vi "Tinius Olsen Output Converter.vi"(8 "error in (no error)":errorcluster, 10 "Data Type (FLOAT)":enum16{"FLOAT", "INT", "BYTE", "SHORT"}(ring), 11 "Data String":string="89C1FC42") -> (0 "error out":errorcluster, 2 "Byte Count":i32=8, 3 "Numeric Conversion - SGL":sgl=126.378)   [LabVIEW 2013]
doc: "This subVI converts ASCII Hex data returned from the Tinius Olsen Model 398 Display device to standard numeric values. Byte reversal is performed within the subVI as appropriate. Only the following data encodings are supported for the 398 Display (Packed Binary Format is not included):\n\nFLOAT = 32-bit (single-precision) floating point number (8 characters),\nINT = 16-bit integer (4 characters),\nBYTE = 8-bit integer (2 characters),\nSHORT = 4-bit integer (1 character).\n\nFor simplicity, all converted values are returned as single precision data type (SGL), even in the case of expected integers. Integer data types are assumed to be unsigned. For more details, please see: people.rit.edu/jdweme/labview/Tinius Olsen Data Conversion.pdf\n\nJohn D. Wellin\nDept. of Mechanical Engineering\nRochester Institute of Technology\nJames E. Gleason Bldg. 09-2014\n76 Lomb Memorial Drive\nRochester, NY 14623-5604\nOffice: 585-475-5223\nFax: 585-475-7710\nEmail: jdweme@rit.edu\nWeb: people.rit.edu/jdweme"
uses:
  <vilib>/regexp/Match Regular Expression.xnode
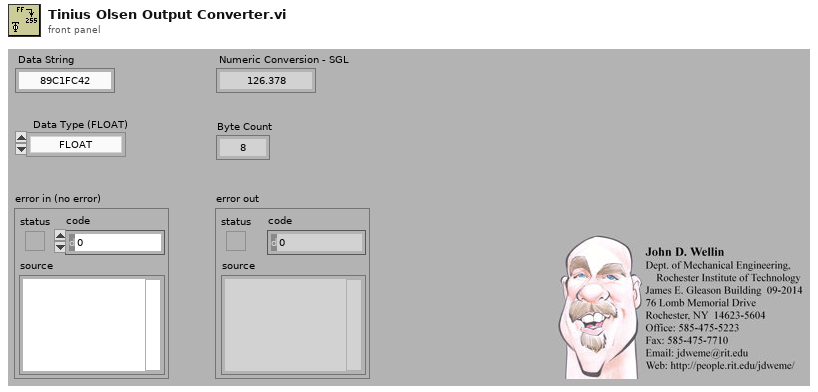
[diagram p1: front panel]
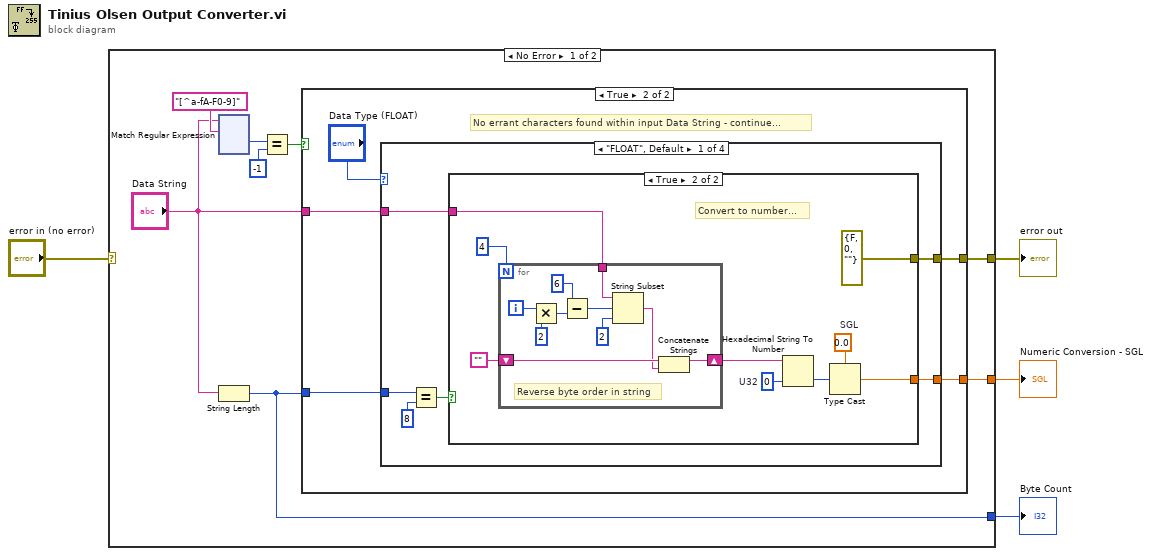
[diagram p0: block diagram]
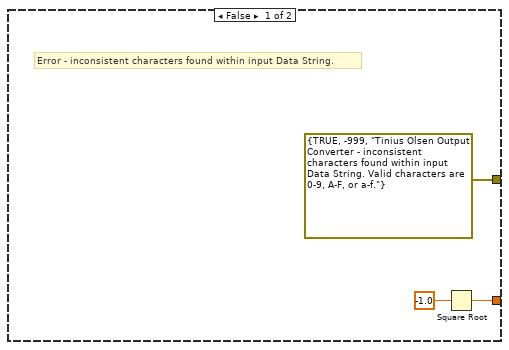
[diagram p2: hidden frame]
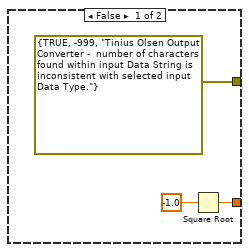
[diagram p3: hidden frame]
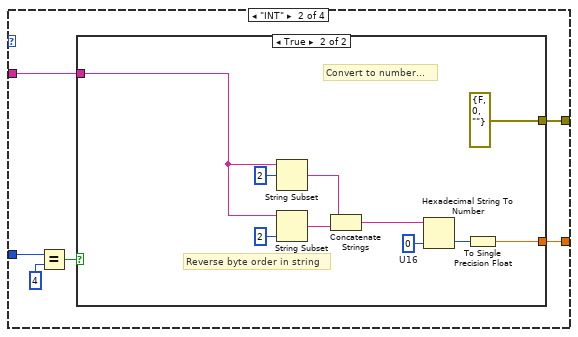
[diagram p4: hidden frame]
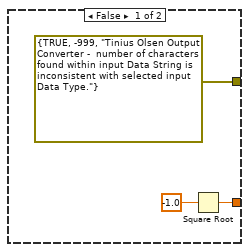
[diagram p5: hidden frame]
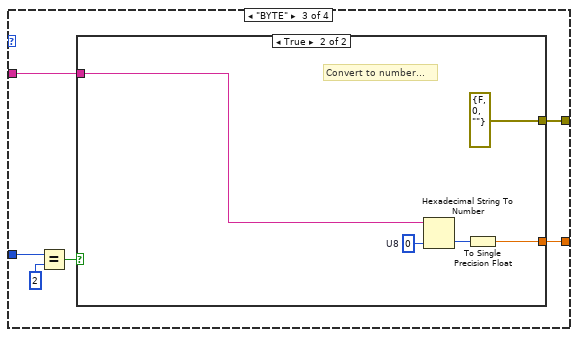
[diagram p6: hidden frame]
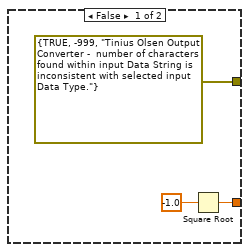
[diagram p7: hidden frame]
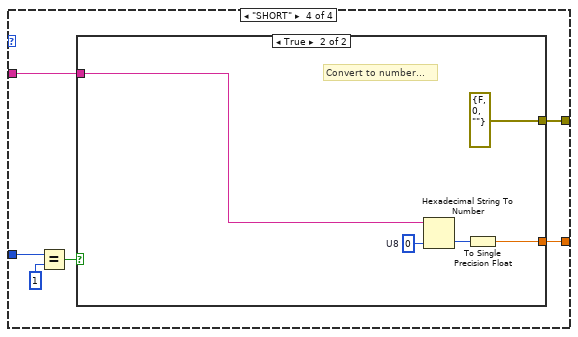
[diagram p8: hidden frame]
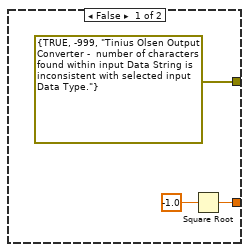
[diagram p9: hidden frame]
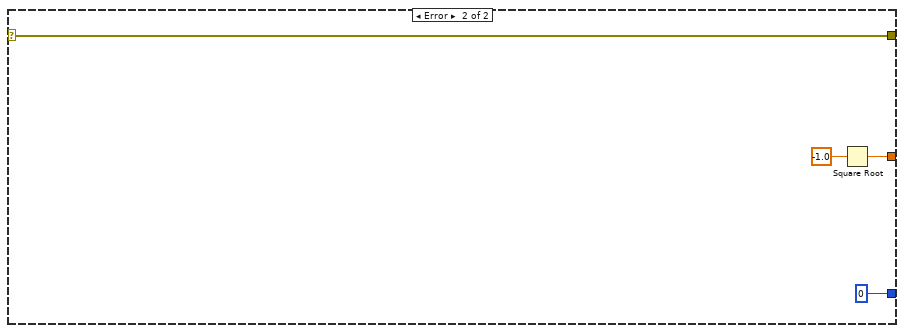
[diagram p10: hidden frame]
diagram:
  n1 = case shown="No Error" "error in (no error)" {
    selector: "error in (no error)" -> [_ w213]
    tunnel: [w11 w211] -> w4
    tunnel: [w7 w213] -> w3
    tunnel: [w5 0] -> w1
    frame No Error {
      n2 = xnode "Match Regular Expression"("input string"="Data String", "regular expression"="[^a-fA-F0-9]") -> ("offset past match"=w10:i32)  [unwired: 4 in, 4 out]
      n3 = String Length(string="Data String") -> (length=w5:i32)
      n4 = Equal?(x=w10, y=-1) -> (x = y?=w8:bool)
      n5 = case shown="True" w8 {
        tunnel: "Data String" -> [_ w18]
        tunnel: [w14 w19] -> w11
        tunnel: [errorcluster {TRUE, -999, "Tinius Olsen Output Converter - inconsistent characters found within input Data String. Valid characters are 0-9, A-F, or a-f."} w17] -> w7
        tunnel: w5 -> [_ w16]
        frame False {
          # "Error - inconsistent characters found within input Data String."
          n6 = Square Root(x=sgl -1.0) -> (sqrt(x)=w14:sgl)
        }
        frame True {
          # "No errant characters found within input Data String - continue..."
          n7 = case shown="\"FLOAT\", Default" "Data Type (FLOAT)" {
            tunnel: w18 -> [w25 w53 w72 w86]
            tunnel: [w26 w54 w73 w87] -> w19
            tunnel: [w22 w50 w69 w83] -> w17
            tunnel: w16 -> [w21 w49 w68 w82]
            frame "FLOAT", Default {
              n8 = Equal?(x=w21, y=8) -> (x = y?=w23:bool)
              n9 = case shown="True" w23 {
                tunnel: [w27 w32] -> w26
                tunnel: w25 -> [_ w31]
                tunnel: [errorcluster {TRUE, -999, "Tinius Olsen Output Converter -  number of characters found within input Data String is inconsistent with selected input Data Type."} errorcluster {FALSE, 0, ""}] -> w22
                frame False {
                  n10 = Square Root(x=sgl -1.0) -> (sqrt(x)=w27:sgl)
                }
                frame True {
                  w33 = u32 0  # U32
                  w38 = sgl 0.0  # SGL
                  # "Convert to number..."
                  n11 = for {
                    N: 4 -> [_]
                    tunnel: w31 -> [w48]
                    shift-right: [w39] -> w35
                    shift-left: "" -> [w41]
                    i -> [w44]
                    # "Reverse byte order in string"
                    n12 = Multiply(x=w44, y=2 ("x")) -> (x*y=w43:i32)
                    n13 = Subtract(x=6, y=w43) -> (x-y=w46:i32)
                    n14 = String Subset(string=w48, offset (0)=w46, length (rest)=2 ("length (rest)")) -> (substring=w40:string)
                    n15 = Concatenate Strings(w41, w40) -> (w39:string)
                  }
                  n16 = Hexadecimal String To Number(string=w35, default (0uL)=w33) -> (number=w34:u32)  [unwired: 1 in, 1 out]
                  n17 = Type Cast(type=w38, x=w34) -> (*(type *) &x=w32:sgl)
                }
              }
            }
            frame "INT" {
              n18 = Equal?(x=w49, y=4) -> (x = y?=w51:bool)
              n19 = case shown="True" w51 {
                tunnel: [w55 w59] -> w54
                tunnel: w53 -> [_ w58]
                tunnel: [errorcluster {TRUE, -999, "Tinius Olsen Output Converter -  number of characters found within input Data String is inconsistent with selected input Data Type."} errorcluster {FALSE, 0, ""}] -> w50
                frame False {
                  n20 = Square Root(x=sgl -1.0) -> (sqrt(x)=w55:sgl)
                }
                frame True {
                  w66 = u16 0  # U16
                  # "Reverse byte order in string"
                  # "Convert to number..."
                  n21 = String Subset(string=w58, offset (0)=2 ("length (rest)")) -> (substring=w62:string)  [unwired: 1 in]
                  n22 = String Subset(string=w58, length (rest)=2 ("length (rest)")) -> (substring=w61:string)  [unwired: 1 in]
                  n23 = Concatenate Strings(w62, w61) -> (w65:string)
                  n24 = Hexadecimal String To Number(string=w65, default (0uL)=w66) -> (number=w60:u16)  [unwired: 1 in, 1 out]
                  n25 = To Single Precision Float(number=w60) -> (single precision float=w59:sgl)
                }
              }
            }
            frame "BYTE" {
              n26 = Equal?(x=w68, y=2) -> (x = y?=w70:bool)
              n27 = case shown="True" w70 {
                tunnel: [w74 w78] -> w73
                tunnel: w72 -> [_ w77]
                tunnel: [errorcluster {TRUE, -999, "Tinius Olsen Output Converter -  number of characters found within input Data String is inconsistent with selected input Data Type."} errorcluster {FALSE, 0, ""}] -> w69
                frame False {
                  n28 = Square Root(x=sgl -1.0) -> (sqrt(x)=w74:sgl)
                }
                frame True {
                  w80 = u8 0  # U8
                  # "Convert to number..."
                  n29 = Hexadecimal String To Number(string=w77, default (0uL)=w80) -> (number=w79:u8)  [unwired: 1 in, 1 out]
                  n30 = To Single Precision Float(number=w79) -> (single precision float=w78:sgl)
                }
              }
            }
            frame "SHORT" {
              n31 = Equal?(x=w82, y=1) -> (x = y?=w84:bool)
              n32 = case shown="True" w84 {
                tunnel: [w88 w92] -> w87
                tunnel: w86 -> [_ w91]
                tunnel: [errorcluster {TRUE, -999, "Tinius Olsen Output Converter -  number of characters found within input Data String is inconsistent with selected input Data Type."} errorcluster {FALSE, 0, ""}] -> w83
                frame False {
                  n33 = Square Root(x=sgl -1.0) -> (sqrt(x)=w88:sgl)
                }
                frame True {
                  w94 = u8 0  # U8
                  # "Convert to number..."
                  n34 = Hexadecimal String To Number(string=w91, default (0uL)=w94) -> (number=w93:u8)  [unwired: 1 in, 1 out]
                  n35 = To Single Precision Float(number=w93) -> (single precision float=w92:sgl)
                }
              }
            }
          }
        }
      }
    }
    frame Error {
      n36 = Square Root(x=sgl -1.0) -> (sqrt(x)=w211:sgl)
    }
  }
  "Numeric Conversion - SGL" <- w4
  "error out" <- w3
  "Byte Count" <- w1
